vi "Main.vi"(7 "Actor Layer":refnum<class "Actor Layer.lvclass">, 11 "Actor":T1) -> (3 "Actor":T1, 4 "Error":errorcluster, 5 "Actor Layer":refnum<class "Actor Layer.lvclass">)   [LabVIEW 2020, in "_Template.lvlib" / "{{Actor}}.lvlib" / "Actor Layer.lvclass"]
uses:
  Actor Layer.lvclass
  Actor Layer.lvclass/Actor Layer.ctl
  C:/Users/nathan.davis/Desktop/personal/jettl-harness/repos/jettl/src/jettl Tools/_Template/{{Actor}}/Actor Layer/Actor Layer.lvclass
  C:/Users/nathan.davis/Desktop/personal/jettl-harness/repos/jettl/src/jettl Tools/_Template/{{Msg}}/Actor Msg/Actor Msg.lvclass
  C:/Users/nathan.davis/Desktop/personal/jettl-harness/repos/jettl/src/jettl/jettl/Actor Layer/Actor Layer.lvclass
  jettl/jettl/jettl.lvlib
  jettl/jettl/Msg/Msg.lvclass
  jettl/jettl/Origin.ctl
  jettl/jettl/Lifecycle.ctl
  jettl/jettl/Msg Attribs.ctl
  jettl/jettl/Msg.ctl
  jettl/jettl/Post Setup.ctl
  jettl/jettl/Pre Setup.ctl
  jettl/jettl/Msg Set.ctl
  jettl/jettl/Actor Attribs.ctl
  jettl/jettl/Children.ctl
  jettl/jettl/Actor.ctl
  jettl/jettl/Layer Type.ctl
  jettl/jettl/Layer Attribs.ctl
  jettl/jettl/Layer Map.ctl
  jettl/jettl/Actor Layer/Actor Layer.lvclass
  jettl/jettl/Implemented Map.ctl
types:
  T1 = typedef "jettl.lvlib/Actor.ctl" = cluster{"Self":T2, "Parent":T2, "Children":T9}
  T2 = typedef "jettl.lvlib/Actor Attribs.ctl" = cluster{"Alias":string, "Msg Set":T3, "Root":bool, "Msg DVR Event":refnum<user-event>, "Msg DVR Event Ref":refnum<event-registration>, "Pre Setup Queue":refnum<queue>, "Begin Setup Queue":refnum<queue>, "Post Setup Queue":refnum<queue>, "Begin Loop Queue":refnum<queue>, "VI Ref":refnum<vi>, "Destroy Queue":refnum<queue>, "Lifecycle":T4, "Current Layer Index":i32, "Layer Map":T5, "Implemented Map":T8}
  T3 = typedef "jettl.lvlib/Msg Set.ctl" = set{refnum<class "Msg.lvclass">}
  T4 = typedef "jettl.lvlib/Lifecycle.ctl" = enum16{"Initializing", "Setting Up", "Starting", "Running", "Stopping", "Tearing Down", "Terminated"}
  T5 = typedef "jettl.lvlib/Layer Map.ctl" = map{i32, T6}
  T6 = typedef "jettl.lvlib/Layer Attribs.ctl" = cluster{"Msg Set":T3, "Layer Type":T7, "Actor Layer":refnum<class "Actor Layer.lvclass">}
  T7 = typedef "jettl.lvlib/Layer Type.ctl" = enum16{"Base", "InnerGlobal", "InnerLocal", "Outer"}
  T8 = typedef "jettl.lvlib/Implemented Map.ctl" = map{refnum<class>, refnum<class "Actor Layer.lvclass">[]}
  T9 = typedef "jettl.lvlib/Children.ctl" = map{string, T2}
  T10 = cluster{"Msg DVR Event Ref":refnum<event-registration>}
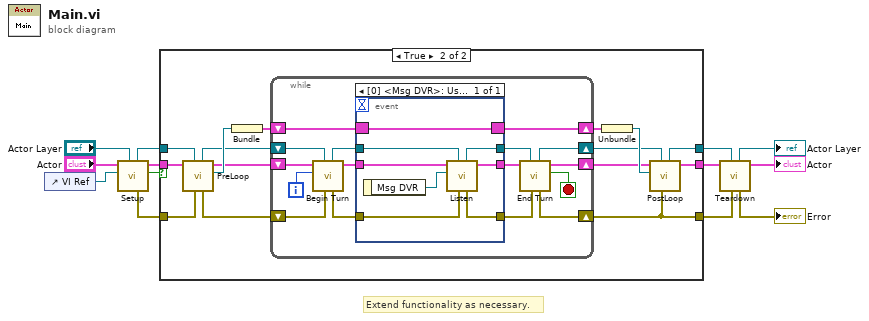
[diagram p0: block diagram]
diagram:
  # "Extend functionality as necessary."
  n1 = control-ref of="VI Ref"() -> (w5:refnum<vi>)
  n2 = call "Setup.vi"(7:"Actor"="Actor Layer", "VIRef"=w5, 11:"Actor"="Actor") -> ("BeginLoop"=w9:bool, 3:"Actor"=w13:T1, "Error"=w12:errorcluster, 5:"Actor"=w7:refnum<class "Actor Layer.lvclass">)  [unwired: 5 in]
  n3 = case shown="True" w9 {
    tunnel: [w16 w25] -> w11
    tunnel: w13 -> [w16 w19]
    tunnel: [w15 w24] -> w10
    tunnel: w12 -> [w15 w18]
    tunnel: w7 -> [w14 w20]
    tunnel: [w14 w21] -> w6
    frame False {
    }
    frame True {
      n4 = call "PreLoop.vi"("Error"=w18, 7:"Actor"=w20, 11:"Actor"=w19) -> ("Msg DVR Event Ref"=w31:refnum<event-registration>, 3:"Actor"=w27:T1, "Error"=w17:errorcluster, 5:"Actor"=w23:refnum<class "Actor Layer.lvclass">)  [unwired: 5 in]
      n5 = Bundle("Msg DVR Event Ref"=w31) -> (w29:T10)  [unwired: 1 in]
      n6 = while {
        shift-right: [w43] -> w26
        shift-left: w27 -> [w36]
        shift-right: [w41] -> w28
        shift-left: w29 -> [w42]
        shift-right: [w45] -> w24
        shift-left: w17 -> [w34]
        shift-right: [w39] -> w22
        shift-left: w23 -> [w38]
        i -> [w32]
        stop <- w47 stop-if-true
        n7 = call "Begin Turn.vi"("Error"=w34, 7:"Actor"=w38, "Iteration"=w32, 11:"Actor"=w36) -> (3:"Actor"=w35:T1, "Error"=w33:errorcluster, 5:"Actor"=w37:refnum<class "Actor Layer.lvclass">)  [unwired: 5 in]
        n8 = event shown="[0] <Msg DVR>: User Event" {
          selector: w42 -> [w48]
          dyn-events: [w48] -> w41
          timeout: _ -> [_]
          tunnel: w35 -> [w52]
          tunnel: [w53] -> w44
          tunnel: [w49] -> w46
          tunnel: w33 -> [w50]
          tunnel: w37 -> [w55]
          tunnel: [w54] -> w40
          event User Event {
            n9 = event-data() -> ("Msg DVR"=w51:refnum<data-value>)  [unwired: 1 in]
            n10 = call "Listen.vi"("Error"=w50, 7:"Actor"=w55, "Msg DVR"=w51, 11:"Actor"=w52) -> (3:"Actor"=w53:T1, "Error"=w49:errorcluster, 5:"Actor"=w54:refnum<class "Actor Layer.lvclass">)  [unwired: 5 in]
          }
        }
        n11 = call "End Turn.vi"("Error"=w46, 7:"Actor"=w40, 11:"Actor"=w44) -> ("Teardown"=w47:bool, 3:"Actor"=w43:T1, "Error"=w45:errorcluster, 5:"Actor"=w39:refnum<class "Actor Layer.lvclass">)  [unwired: 5 in]
      }
      n12 = Unbundle(w28) -> ("Msg DVR Event Ref"=w30:refnum<event-registration>)
      n13 = call "PostLoop.vi"("Error"=w24, 7:"Actor"=w22, "Msg DVR Event Ref"=w30, 11:"Actor"=w26) -> (3:"Actor"=w25:T1, 5:"Actor"=w21:refnum<class "Actor Layer.lvclass">)  [unwired: 6 in]
    }
  }
  n14 = call "Teardown.vi"("Error"=w10, 7:"Actor"=w6, 11:"Actor"=w11) -> (3:"Actor"=→"Actor":T1, "Error"=→"Error":errorcluster, 5:"Actor"=→"Actor Layer":refnum<class "Actor Layer.lvclass">)  [unwired: 6 in]
